vi "Full front panel JJCH2(SubVI).vi"(0 "Signal in":dbl[](array[numeric]), 1 "Time in":dbl[](array[numeric]), 2 "Integrate Array":dbl[](array[numeric]), 3 "Path 1":path, 4 "XYGraph Refnum":refnum<vi>, 6 "Boolean":bool[](array[boolean]), 7 "Add element 1":string, 10 "String":refnum<vi>, 11 "Sample list":i32(listbox)=-1, 12 "Sample list 2":refnum<vi>, 13 "mean In":dbl, 16 "Elapsed Time (s)":dbl) -> (5 "Concentrations":dbl[](array[numeric]), 8 "?":cluster{"all rows":dbl[], "all rows":dbl[]}(graph), 9 "Mean":dbl, 14 "Signal out":dbl[](array[numeric]), 15 "Time out":dbl[](array[numeric]), 17 "Plot":cluster{dbl[], dbl[]}(graph), 18 "Current Element":string, 19 "All samples":i32)   [LabVIEW 2014]
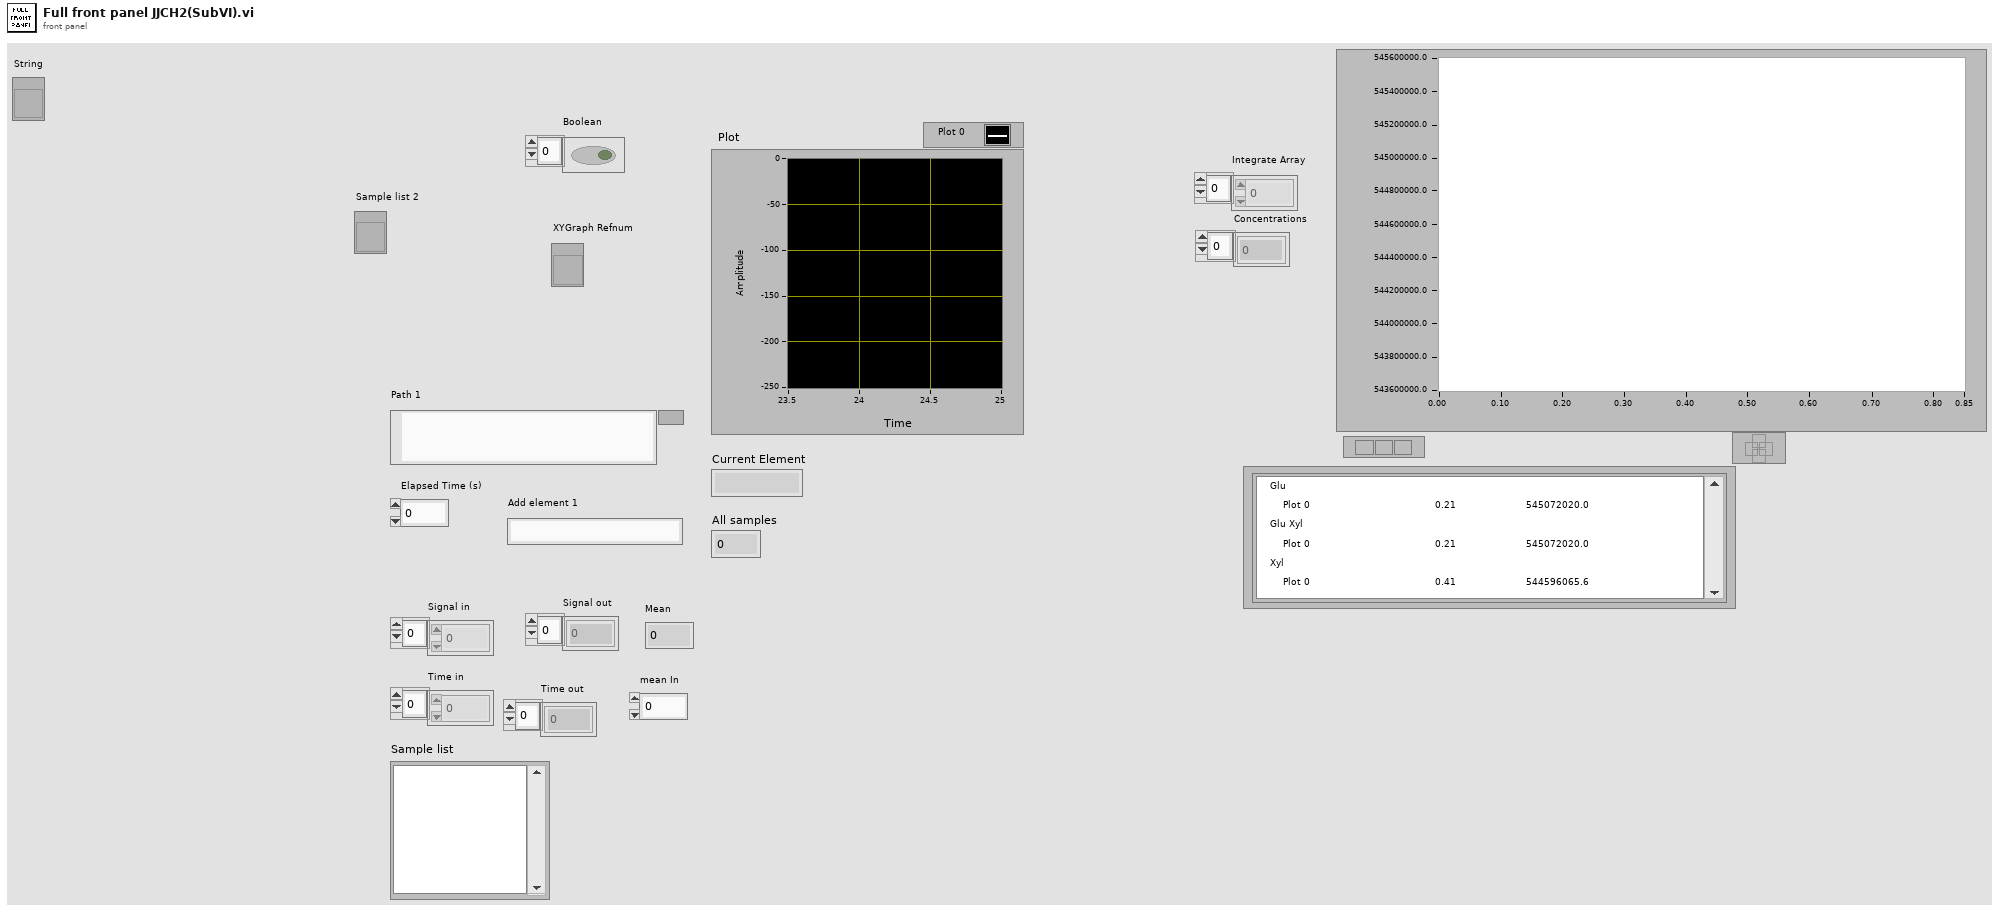
[diagram p1: front panel]
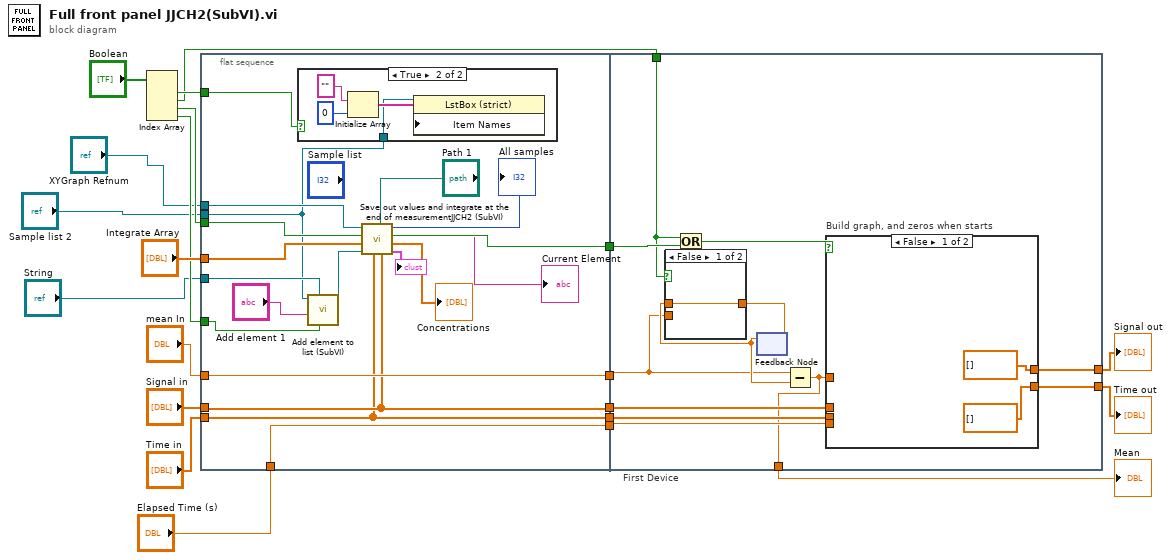
[diagram p0: block diagram]
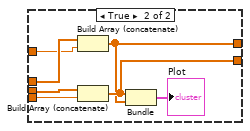
[diagram p4: hidden frame]
diagram:
  n1 = Index Array(array="Boolean") -> (element #1=w7:bool, element #2=w6:bool, element #3=w5:bool, element #4=w4:bool)  [unwired: 4 in]
  n2 = flat-sequence "First Device" {
    tunnel: w5 -> [w31]
    tunnel: "Signal in" -> [w23]
    tunnel: "Time in" -> [w22]
    tunnel: [w23] -> w21
    tunnel: [w22] -> w20
    tunnel: [w36] -> w19
    tunnel: "mean In" -> [w38]
    tunnel: [w38] -> w18
    tunnel: [w31] -> w12
    tunnel: "Elapsed Time (s)" -> [w36]
    tunnel: "Integrate Array" -> [w30]
    tunnel: w7 -> [w35]
    tunnel: w4 -> [w34]
    tunnel: "Sample list 2" -> [w29]
    tunnel: "String" -> [w33]
    tunnel: "XYGraph Refnum" -> [w32]
    tunnel: [w54] -> w16
    tunnel: [w53] -> w17
    tunnel: w21 -> [w52]
    tunnel: w20 -> [w51]
    tunnel: w19 -> [w50]
    tunnel: w18 -> [w45]
    tunnel: w12 -> [w46]
    tunnel: [w44] -> w10
    tunnel: w6 -> [w43]
    frame #0 {
      n3 = case shown="True" w35 {
        tunnel: w29 -> [_ w39]
        frame False {
        }
        frame True {
          n4 = Initialize Array("", 0 ("dimension size")) -> (w42:string[])
          n5 = property on="Property Node" class="LstBox (strict)"(reference=w39, "Item Names"=w42) -> ()  [unwired: 1 in, 2 out]
        }
      }
      n6 = call "Add element to list (SubVI).vi"("Boolean"=w34, "String"=w33, "Add string"="Add element 1", "ListBox in"=w29) -> ()  [unwired: 8 in]
      n7 = call "Save out values and integrate at the end of measurementJJCH2 (SubVI).vi"("Measurement Array"=w23, "Path"="Path 1", "Time Array"=w22, "ListBox in 2"=w29, "Integrate Array"=w30, "Measurement running?"=w31, "XYGraph Refnum"=w32) -> (0:→"?":cluster{"all rows":dbl[], "all rows":dbl[]}, "Concentrations"=→"Concentrations":dbl[], "element"=→"Current Element":string, "size(s)"=→"All samples":i32)  [unwired: 1 in]
    }
    frame #1 {
      n8 = Or(x=w43, y=w46) -> (x .or. y?=w47:bool)
      n9 = feedback #1() -> (w48:dbl)  [unwired: 1 in]
      n10 = case shown="False" w43 {
        tunnel: w45 -> [_ w56]
        tunnel: [w55 w56] -> w49
        tunnel: w48 -> [w55 _]
        frame False {
        }
        frame True {
        }
      }
      n11 = feedback-in #1(w49) -> ()
      n12 = Subtract(x=w45, y=w48) -> (x-y=w44:dbl)
      n13 = case "Build graph, and zeros when starts" shown="False" w47 {
        tunnel: [dbl[] [] w63] -> w53
        tunnel: w52 -> [_ w61]
        tunnel: w51 -> [_ w65]
        tunnel: [dbl[] [] w64] -> w54
        tunnel: w50 -> [_ w62]
        tunnel: w44 -> [_ w60]
        frame False {
        }
        frame True {
          n14 = Build Array (concatenate)(w61, w60) -> (w63:dbl[])
          n15 = Build Array (concatenate)(w65, w62) -> (w64:dbl[])
          n16 = Bundle(w64, w63) -> (→"Plot":cluster{dbl[], dbl[]})  [unwired: 1 in]
        }
      }
    }
  }
  "Signal out" <- w17
  "Time out" <- w16
  "Mean" <- w10
